vi "LED Controls2.vi"(2 "Enum":enum16{"Start", "Run", "End"}(ring)) -> ()   [LabVIEW 2014]
uses:
  TypeDefs/Digital Module 1.ctl
  <vilib>/Rock Robotics/SystemInterfaces/Typedef/FPGA_TypedefDigitalModule.ctl
  <vilib>/Rock Robotics/SystemInterfaces/DIO/FPGA_DIOChannel.ctl
  Team Code/Robot Global Data.vi
panel:
  in  "Digital Module A":T1={"Module"=enum."Digital Module 1", "L Encoder A"=enum."DIO 1", "L Encoder B"=enum."DIO 2", "R Encoder A"=enum."DIO 3", "R Encoder B"=enum."DIO 4", "Compressor"=enum."DIO 5", "Shooter Limit"=enum."DIO 6", "LED 1"=enum."DIO 7", "LED 2"=enum."DIO 8", "LED 3"=enum."DIO 9", "LED 4"=enum."DIO 9", "Shooter Limit 2"=enum."DIO 11", "Unassigned"=enum."DIO 12", "Unassigned"=enum."DIO 13", "Unassigned"=enum."DIO 14"}
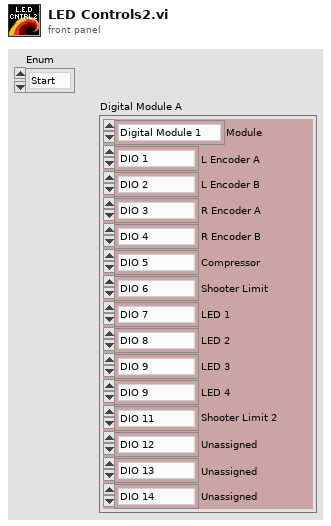
[diagram p1: front panel]
types:
  T1 = typedef "Digital Module 1.ctl" = cluster{"Module":T2, "L Encoder A":T3, "L Encoder B":T3, "R Encoder A":T3, "R Encoder B":T3, "Compressor":T3, "Shooter Limit":T3, "LED 1":T3, "LED 2":T3, "LED 3":T3, "LED 4":T3, "Shooter Limit 2":T3, "Unassigned":T3, "Unassigned":T3, "Unassigned":T3}
  T2 = typedef "FPGA_TypedefDigitalModule.ctl" = enum16{"Digital Module 1", "Digital Module 2"}
  T3 = typedef "FPGA_DIOChannel.ctl" = enum8{"DIO 1", "DIO 2", "DIO 3", "DIO 4", "DIO 5", "DIO 6", "DIO 7", "DIO 8", "DIO 9", "DIO 10", "DIO 11", "DIO 12", "DIO 13", "DIO 14", "Invalid"}
  T4 = enum16{"Nothing", "Load", "Lock", "Pass", "Grab", "Loader Down", "Shoot", "Auto Start", "Tele Start"}
  T5 = typedef "WPI_DigitalOutputDevRef.ctl" = cluster{"Digital Module":T2, "DIO Channel":T3, "DevStatus":errorcluster}
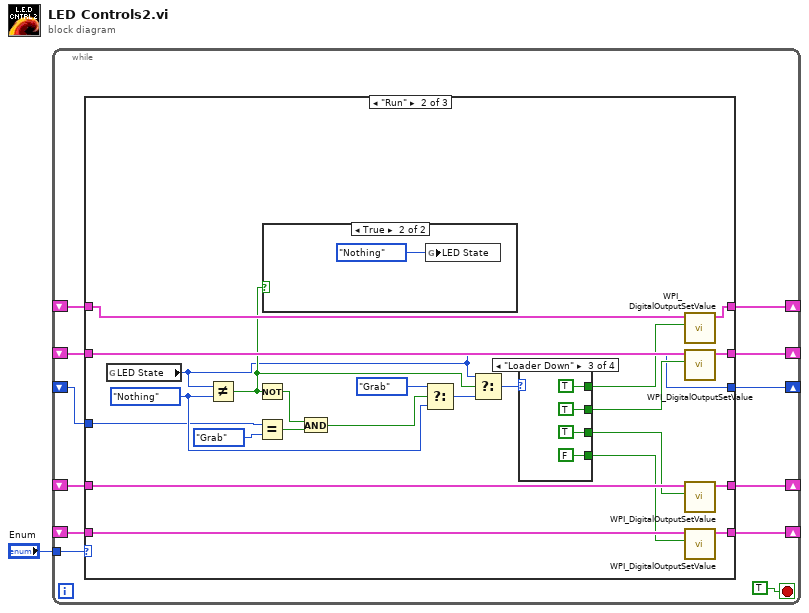
[diagram p0: block diagram]
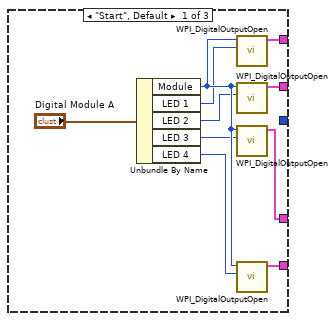
[diagram p2: hidden frame]
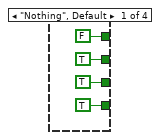
[diagram p4: hidden frame]
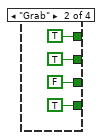
[diagram p5: hidden frame]
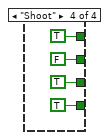
[diagram p6: hidden frame]
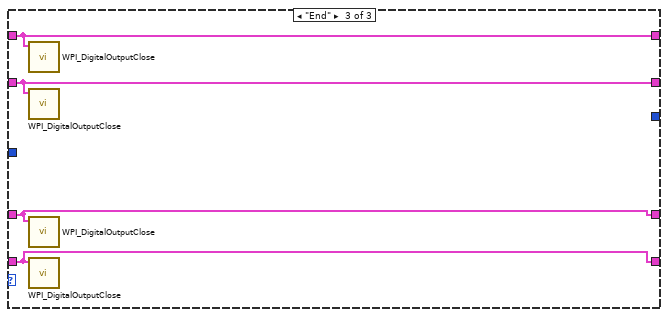
[diagram p7: hidden frame]
diagram:
  n1 = while {
    tunnel: "Enum" -> [w12]
    shift-right: [w10] -> _
    shift-left: _ -> [w11]
    shift-right: [w9] -> _
    shift-left: _ -> [w6]
    shift-right: [w8] -> _
    shift-left: _ -> [w5]
    shift-right: [w7] -> _
    shift-left: _ -> [w4]
    shift-right: [w3] -> _
    shift-left: _ -> [w2]
    stop <- TRUE stop-if-true
    n2 = case shown="\"Run\"" w12 {
      tunnel: w11 -> [_ w42 w64]
      tunnel: [w22 w46 w64] -> w10
      tunnel: [w21 w45 w65] -> w9
      tunnel: [w20 w44 w66] -> w8
      tunnel: [w19 w43 w67] -> w7
      tunnel: w6 -> [_ w41 w65]
      tunnel: w5 -> [_ w40 w66]
      tunnel: w4 -> [_ w39 w67]
      tunnel: [_ w25 _] -> w3
      tunnel: w2 -> [_ w24 _]
      frame "Start", Default {
        n3 = Unbundle By Name("Digital Module A") -> ("Module"=w18:T2, "LED 1"=w14:T3, "LED 2"=w15:T3, "LED 3"=w16:T3, "LED 4"=w17:T3)
        n4 = call <vilib>:"WPI_DigitalOutputOpen.vi"("DIO Channel"=w14, "Digital Module (Module 1)"=w18) -> ("DigitalOutputDevRef"=w22:T5)  [unwired: 8 in, 1 out]
        n5 = call <vilib>:"WPI_DigitalOutputOpen.vi"("DIO Channel"=w15, "Digital Module (Module 1)"=w18) -> ("DigitalOutputDevRef"=w21:T5)  [unwired: 8 in, 1 out]
        n6 = call <vilib>:"WPI_DigitalOutputOpen.vi"("DIO Channel"=w16, "Digital Module (Module 1)"=w18) -> ("DigitalOutputDevRef"=w20:T5)  [unwired: 8 in, 1 out]
        n7 = call <vilib>:"WPI_DigitalOutputOpen.vi"("DIO Channel"=w17, "Digital Module (Module 1)"=w18) -> ("DigitalOutputDevRef"=w19:T5)  [unwired: 8 in, 1 out]
      }
      frame "Run" {
        w27 = T4."Nothing" ("f")
        n8 = global read "Robot Global Data.vi" "LED State"() -> (w25:T4)
        n9 = Not Equal?(x=w25, y=w27) -> (x != y?=w32:bool)
        n10 = Not(x=w32) -> (.not. x?=w31:bool)
        n11 = Equal?(x=w24, y=T4."Grab") -> (x = y?=w30:bool)
        n12 = case shown="True" w32 {
          frame False {
          }
          frame True {
            n13 = global write "Robot Global Data.vi" "LED State"(T4."Nothing" ("f")) -> ()
          }
        }
        n14 = And(x=w31, y=w30) -> (x .and. y?=w28:bool)
        n15 = Select(t=T4."Grab", s=w28, f=w27) -> (s? t:f=w29:T4)
        n16 = Select(t=w25, s=w32, f=w29) -> (s? t:f=w33:T4)
        n17 = case shown="\"Loader Down\"" w33 {
          tunnel: [FALSE TRUE TRUE TRUE] -> w38
          tunnel: [TRUE TRUE TRUE FALSE] -> w37
          tunnel: [TRUE FALSE TRUE TRUE] -> w36
          tunnel: [TRUE TRUE FALSE TRUE] -> w35
          frame "Nothing", Default {
          }
          frame "Grab" {
          }
          frame "Loader Down" {
          }
          frame "Shoot" {
          }
        }
        n18 = call <vilib>:"WPI_DigitalOutputSetValue.vi"("Value"=w38, "DigitalOutputDevRef"=w42) -> ("DigitalOutputDevRef"=w46:T5)  [unwired: 8 in, 1 out]
        n19 = call <vilib>:"WPI_DigitalOutputSetValue.vi"("Value"=w37, "DigitalOutputDevRef"=w41) -> ("DigitalOutputDevRef"=w45:T5)  [unwired: 8 in, 1 out]
        n20 = call <vilib>:"WPI_DigitalOutputSetValue.vi"("Value"=w36, "DigitalOutputDevRef"=w40) -> ("DigitalOutputDevRef"=w44:T5)  [unwired: 8 in, 1 out]
        n21 = call <vilib>:"WPI_DigitalOutputSetValue.vi"("Value"=w35, "DigitalOutputDevRef"=w39) -> ("DigitalOutputDevRef"=w43:T5)  [unwired: 8 in, 1 out]
      }
      frame "End" {
        n22 = call <vilib>:"WPI_DigitalOutputClose.vi"("DigitalOutputDevRef"=w64) -> ()  [unwired: 10 in, 1 out]
        n23 = call <vilib>:"WPI_DigitalOutputClose.vi"("DigitalOutputDevRef"=w65) -> ()  [unwired: 10 in, 1 out]
        n24 = call <vilib>:"WPI_DigitalOutputClose.vi"("DigitalOutputDevRef"=w66) -> ()  [unwired: 10 in, 1 out]
        n25 = call <vilib>:"WPI_DigitalOutputClose.vi"("DigitalOutputDevRef"=w67) -> ()  [unwired: 10 in, 1 out]
      }
    }
  }
